vi "ESC_Harness_InstructionsListener.vi"(7 "error in (no error)":errorcluster, 10 "Input":T1={"Test_File"="", "Status"="OK", "RF_Center_Freq"="0", "RF_Gain"="0", "BB_Gain"="0", "Error"=""}) -> (0 "error out":errorcluster)   [LabVIEW 2016]
uses:
  <vilib>/httpClient/POSTBuffer.vi
  <vilib>/httpClient/LabVIEWHTTPClient.lvlib
panel:
  # "Use the Web Service Request input terminal to call the VIs on the Web Services palette. Do not remove it from the connector pane unless you don't need access to the palette."
  # "Each additional control wired to the connector pane will be available as an input in the URL. To include an indicator in terminal-mode output (the default setting), it must also be wired to the connector pane."
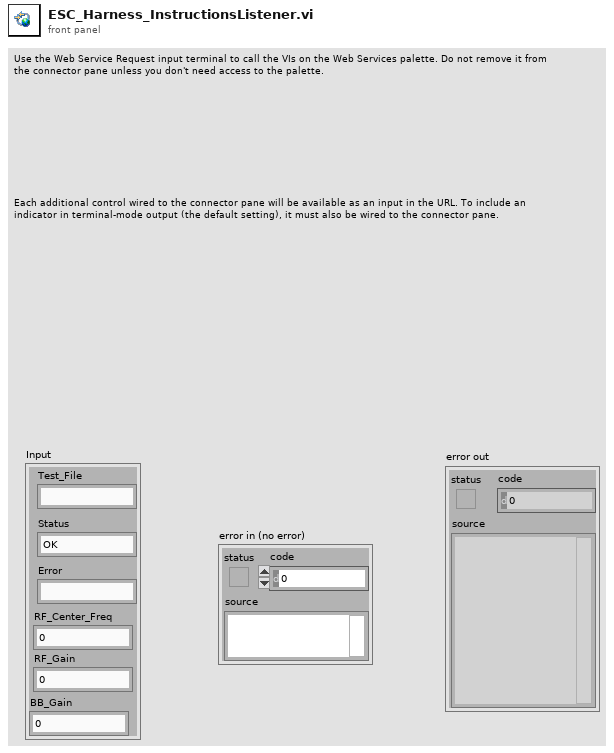
[diagram p1: front panel]
types:
  T1 = cluster{"Test_File":string, "Status":string, "RF_Center_Freq":string, "RF_Gain":string, "BB_Gain":string, "Error":string}
  T2 = typedef "LabVIEWHTTPClient.lvlib/ClientHandle.ctl" = refnum<k1>
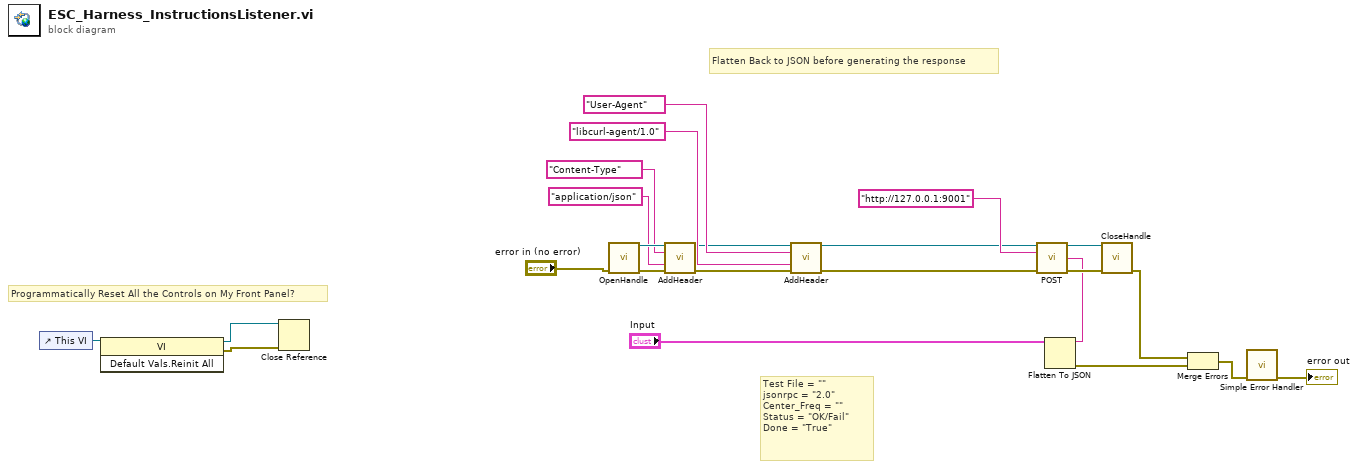
[diagram p0: block diagram]
diagram:
  # "Programmatically Reset All the Controls on My Front Panel?"
  # "Test File = \"\"\njsonrpc = \"2.0\"\nCenter_Freq = \"\"\nStatus = \"OK/Fail\"\nDone = \"True\""
  # "Flatten Back to JSON before generating the response"
  n1 = control-ref of="This VI"() -> (w4:refnum<vi>)
  n2 = invoke class="VI" method="Default Vals.Reinit All"(reference=w4) -> (reference out=w3:refnum<vi>, error out=w2:errorcluster)  [unwired: 2 in, 1 out]
  n3 = Close Reference(reference=w3, error in (no error)=w2) -> ()  [unwired: 1 out]
  n4 = call <vilib>:"OpenHandle.vi"("error in (no error)"="error in (no error)") -> ("client handle out"=w21:T2, "error out"=w20:errorcluster)  [unwired: 13 in]
  n5 = call <vilib>:"AddHeader.vi"("client handle"=w21, "header"="Content-Type", "value"="application/json", "error in (no error)"=w20) -> ("client handle out"=w11:T2, "error out"=w10:errorcluster)  [unwired: 10 in]
  n6 = call <vilib>:"AddHeader.vi"("client handle"=w11, "header"="User-Agent", "value"="libcurl-agent/1.0", "error in (no error)"=w10) -> ("client handle out"=w8:T2, "error out"=w9:errorcluster)  [unwired: 10 in]
  n7 = Flatten To JSON(anything="Input") -> (JSON string=w6:string, 11:w7:errorcluster)  [unwired: 2 in]
  n8 = call-poly <vilib>:"POST.vi"("client handle"=w8, "url"="http://127.0.0.1:9001" ("value"), "buffer"=w6, "error in (no error)"=w9) -> ("client handle out"=w22:T2, "error out"=w23:errorcluster)  [unwired: 8 in, 2 out]
  n9 = call <vilib>:"CloseHandle.vi"("client handle"=w22, "error in (no error)"=w23) -> ("error out"=w15:errorcluster)  [unwired: 13 in]
  n10 = Merge Errors(w15, w7) -> (w14:errorcluster)
  n11 = call <vilib>:"Simple Error Handler.vi"("error in (no error)"=w14) -> ("error out"=→"error out":errorcluster)  [unwired: 4 in, 4 out]
